vi "ToStreamID.vi"(10 "Category":string, 11 "ID in":string) -> (3 "ID out":string)   [LabVIEW 2017]
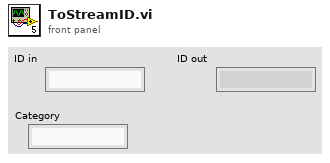
[diagram p1: front panel]
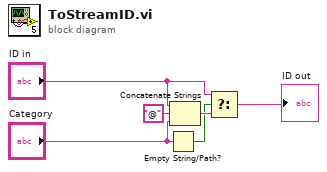
[diagram p0: block diagram]
diagram:
  n1 = Empty String/Path?(string/path="Category") -> (empty?=w3:bool)
  n2 = Concatenate Strings("ID in", "@" ("string"), "Category") -> (w5:string)
  n3 = Select(t="ID in", s=w3, f=w5) -> (s? t:f=→"ID out":string)
